vi "FTW-CodeGen-XNodeUpdateState.vi"(0 "XRef":refnum<vi>, 5 "Previous Version":T1, 11 "error in":errorcluster) -> (6 "Reply":string[](array[string]))   [LabVIEW 2015]
uses:
  FTW-CodeGen-XNodeReplyType.ctl
panel:
  # "Inputs"
  # "Outputs"
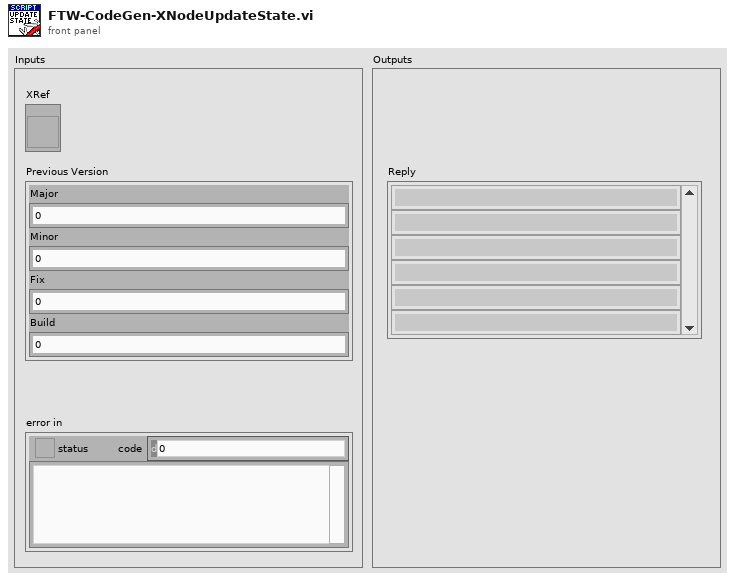
[diagram p1: front panel]
types:
  T1 = cluster{"Major":u16, "Minor":u16, "Fix":u16, "Build":u16}
  T2 = typedef "FTW-CodeGen-XNodeReplyType.ctl" = enum16{"NoReply", "ForceAdaptToInputs", "UpdateTerms", "GenCode", "GenCode+CosmeticUpdate"}
  T3 = cluster{"Major":i32, "Minor":i32, "Fix":i32, "Build":i32}
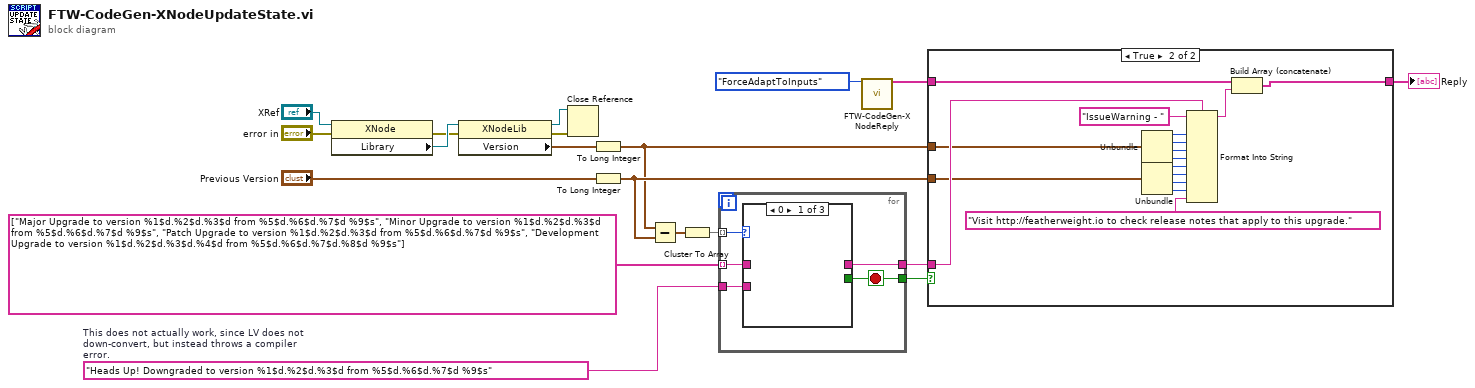
[diagram p0: block diagram]
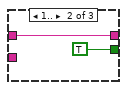
[diagram p2: hidden frame]
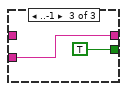
[diagram p3: hidden frame]
diagram:
  w3 = "Heads Up! Downgraded to version %1$d.%2$d.%3$d from %5$d.%6$d.%7$d %9$s"  # This does not actually work, since LV does not down-convert, but instead throws a compiler error.
  n1 = property class="XNode"(reference="XRef", error in="error in") -> (error out=w16:errorcluster, "Library"=w17:refnum<vi>)  [unwired: 1 out]
  n2 = property class="XNodeLib"(reference=w17, error in=w16) -> (reference out=w13:refnum<vi>, error out=w12:errorcluster, "Version"=w1:T1)
  n3 = Close Reference(reference=w13, error in (no error)=w12) -> ()  [unwired: 1 out]
  n4 = To Long Integer(number=w1) -> (32bit integer=w2:T3)
  n5 = To Long Integer(number="Previous Version") -> (32bit integer=w5:T3)
  n6 = Subtract(x=w2, y=w5) -> (x-y=w10:T3)
  n7 = Cluster To Array(cluster=w10) -> (array=w9:i32[])
  n8 = for {
    tunnel: w9 -> [w24] mode=indexing
    tunnel: [w23] -> w7
    tunnel: string[] ["Major Upgrade to version %1$d.%2$d.%3$d from %5$d.%6$d.%7$d %9$s", "Minor Upgrade to version %1$d.%2$d.%3$d from %5$d.%6$d.%7$d %9$s", "Patch Upgrade to version %1$d.%2$d.%3$d from %5$d.%6$d.%7$d %9$s", "Development Upgrade to version %1$d.%2$d.%3$d.%4$d from %5$d.%6$d.%7$d.%8$d %9$s"] -> [w22] mode=indexing
    tunnel: [w21] -> w4
    tunnel: w3 -> [w20]
    stop <- w21 stop-if-true
    n9 = case shown="0" w24 {
      tunnel: [_ w26 w27] -> w23
      tunnel: w22 -> [_ w26 _]
      tunnel: [_ TRUE TRUE] -> w21
      tunnel: w20 -> [_ _ w27]
      frame 0 {
      }
      frame 1.. {
      }
      frame ..-1 {
      }
    }
  }
  n10 = call "FTW-CodeGen-XNodeReply.vi"("XNode Reply Type"=FTW-CodeGen-XNodeReplyType."ForceAdaptToInputs") -> ("Reply"=w15:string[])  [unwired: 14 in]
  n11 = case shown="True" w4 {
    tunnel: w15 -> [w29 w45]
    tunnel: [w29 w30] -> w14
    tunnel: w7 -> [_ w35]
    tunnel: w5 -> [_ w34]
    tunnel: w2 -> [_ w33]
    frame False {
    }
    frame True {
      n12 = Unbundle(w33) -> ("Major"=w37:i32, "Minor"=w38:i32, "Fix"=w39:i32, "Build"=w43:i32)
      n13 = Unbundle(w34) -> ("Major"=w40:i32, "Minor"=w41:i32, "Fix"=w42:i32, "Build"=w44:i32)
      n14 = Format Into String(format string=w35, initial string="IssueWarning - ", w37, w38, w39, w43, w40, w41, w42, w44, "Visit http://featherweight.io to check release notes that apply to this upgrade." ("format string")) -> (resulting string=w36:string)  [unwired: 1 in, 1 out]
      n15 = Build Array (concatenate)(w45, w36) -> (w30:string[])
    }
  }
  "Reply" <- w14
